vi "timekeeper get status.vi"() -> (0 "timekeeper locked (g)":bool, 1 "Offset from Timeref (g)":fxp<+/-,21,21>)   [LabVIEW 2011, in "EPS_Timekeeper.lvlib"]
doc: "This provides status on the current state of the FPGA Timekeeper"
uses:
  <vilib>/addons/Electrical Power/Example Support/PMU/Time Keeper/EPS_Timekeeper.lvlib
  <vilib>/addons/Electrical Power/Example Support/PMU/Time Keeper/timekeeper locked (g).vi
  <vilib>/addons/Electrical Power/Example Support/PMU/Time Keeper/timekeeper offset from timeref (g).vi
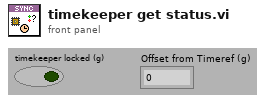
[diagram p1: front panel]
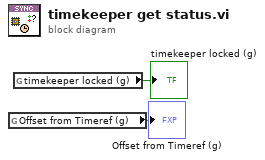
[diagram p0: block diagram]
diagram:
  n1 = global read "timekeeper offset from timeref (g).vi" "Offset from Timeref (g)"() -> (→"Offset from Timeref (g)":fxp<+/-,21,21>)
  n2 = global read "timekeeper locked (g).vi" "timekeeper locked (g)"() -> (→"timekeeper locked (g)":bool)
